vi "FreqC.Read Measurement.vi"(8 "error In":errorcluster, 11 "FreqC Session in":T1) -> (0 "error out":errorcluster, 2 "Measurement":dbl format="%#_12g", 3 "FreqC Session out":T1)   [LabVIEW 2018]
uses:
  typedefs/FreqC.Session.ctl
  <instrlib>/Agilent 532XX Series/Public/Data/Read Measurement (Single).vi
  <instrlib>/Agilent 532XX Series/Agilent 532XX Series.lvlib
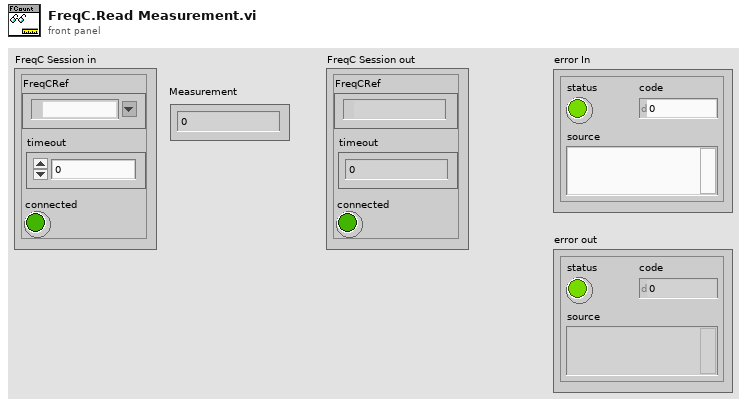
[diagram p1: front panel]
types:
  T1 = typedef "FreqC.Session.ctl" = cluster{"FreqCRef":refnum<visa-resource-name>, "timeout":dbl, "connected":bool}
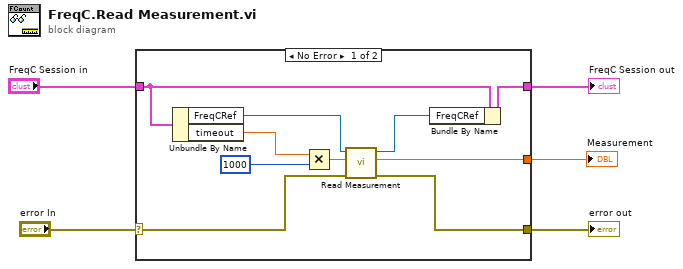
[diagram p0: block diagram]
diagram:
  n1 = case shown="No Error" "error In" {
    selector: "error In" -> [w7 w17]
    tunnel: [w6 w17] -> w4
    tunnel: "FreqC Session in" -> [w15 w16]
    tunnel: [w14 w16] -> w2
    tunnel: [w13 _] -> w1
    frame No Error {
      n2 = Unbundle By Name(w15) -> ("FreqCRef"=w12:refnum<visa-resource-name>, "timeout"=w10:dbl)
      n3 = Multiply(x=w10, y=u32 1000 ("Timeout (10000 ms)")) -> (x*y=w8:dbl)
      n4 = call-poly <instrlib>:"Read Measurement.vi"("error in (no error)"=w7, "Timeout (10000 ms)"=w8, "VISA resource name"=w12) -> ("error out"=w6:errorcluster, "Measurement"=w13:dbl, "VISA resource name out"=w11:refnum<visa-resource-name>)  [unwired: 6 in]
      n5 = Bundle By Name(cluster=w15, "FreqCRef"=w11) -> (w14:T1)
    }
    frame Error {
    }
  }
  "error out" <- w4
  "FreqC Session out" <- w2
  "Measurement" <- w1
